vi "SignalSet.vi"(0 "时间(s)":dbl[](array[numeric]), 1 "数组(u64)":u64[](array[numeric]), 2 "信号配置":cluster{"起始位":u8, "长度":u8, "分辨率":dbl, "偏移量":dbl}={"起始位"=0, "长度"=1, "分辨率"=1.0, "偏移量"=0.0}, 3 "下拉列表":u16(ring) items=["Intel", "Motorola"]) -> (6 "信号":cluster{"时间(s)":dbl[], "数据":dbl[]})   [LabVIEW 2015]
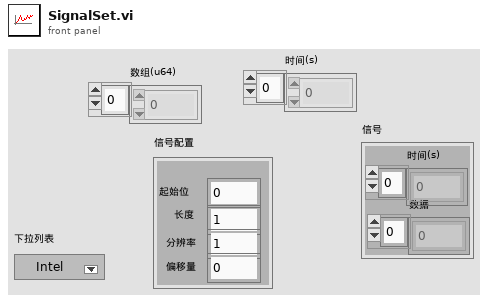
[diagram p1: front panel]
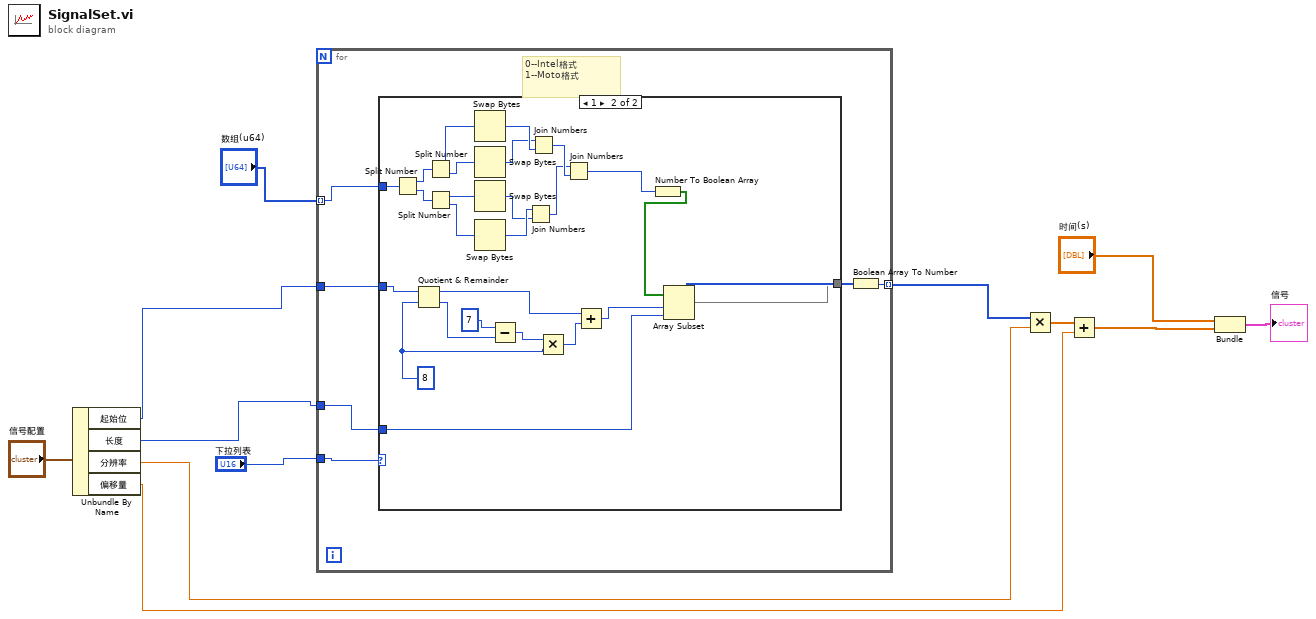
[diagram p0: block diagram]
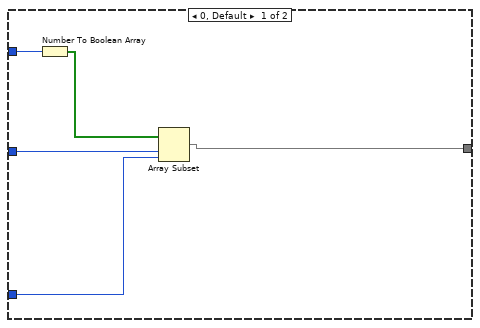
[diagram p2: hidden frame]
diagram:
  n1 = Unbundle By Name("信号配置") -> ("起始位"=w4:u8, "长度"=w3:u8, "分辨率"=w2:dbl, "偏移量"=w1:dbl)
  n2 = for {
    tunnel: "数组(u64)" -> [w13] mode=indexing
    tunnel: w4 -> [w18]
    tunnel: w3 -> [w17]
    tunnel: [w16] -> w7 mode=indexing
    tunnel: "下拉列表" -> [w14]
    # "0--Intel格式\n1--Moto格式"
    n3 = case shown="1" w14 {
      tunnel: w18 -> [w23 w29]
      tunnel: w17 -> [w22 w48]
      tunnel: [w21 w30] -> w15
      tunnel: w13 -> [w20 w47]
      frame 0, Default {
        n4 = Number To Boolean Array(number=w20) -> (Boolean array=w19:bool[])
        n5 = Array Subset(array=w19, index=w23, length=w22) -> (w21:bool[])
      }
      frame 1 {
        w27 = 8
        n6 = Split Number(x=w47) -> (hi(x)=w46:u32, lo(x)=w45:u32)
        n7 = Quotient & Remainder(x=w29, y=w27) -> (x-y*floor(x/y)=w24:i32, floor(x/y)=w28:i32)
        n8 = Split Number(x=w46) -> (hi(x)=w41:u16, lo(x)=w42:u16)
        n9 = Split Number(x=w45) -> (hi(x)=w43:u16, lo(x)=w44:u16)
        n10 = Swap Bytes(anything=w41) -> (byte swapped=w40:u16)
        n11 = Swap Bytes(anything=w42) -> (byte swapped=w39:u16)
        n12 = Swap Bytes(anything=w43) -> (byte swapped=w37:u16)
        n13 = Swap Bytes(anything=w44) -> (byte swapped=w38:u16)
        n14 = Subtract(x=7, y=w28) -> (x-y=w25:i32)
        n15 = Join Numbers(hi=w38, lo=w37) -> ((hi.lo)=w35:u32)
        n16 = Join Numbers(hi=w39, lo=w40) -> ((hi.lo)=w36:u32)
        n17 = Multiply(x=w25, y=w27) -> (x*y=w32:i32)
        n18 = Join Numbers(hi=w35, lo=w36) -> ((hi.lo)=w34:u64)
        n19 = Add(x=w24, y=w32) -> (x+y=w31:i32)
        n20 = Number To Boolean Array(number=w34) -> (Boolean array=w33:bool[])
        n21 = Array Subset(array=w33, index=w31, length=w48) -> (w30:bool[])
      }
    }
    n22 = Boolean Array To Number(Boolean array=w15) -> (number=w16:u32)
  }
  n23 = Multiply(x=w7, y=w2) -> (x*y=w8:dbl[])
  n24 = Add(x=w8, y=w1) -> (x+y=w11:dbl[])
  n25 = Bundle("时间(s)"="时间(s)", w11) -> (→"信号":cluster{"时间(s)":dbl[], dbl[]})  [unwired: 1 in]
